vi "Exo5.vi"() -> ()   [LabVIEW 2018]
panel:
  in  "stop":bool
  in  "Débit":dbl
  out "Tank 2":dbl(slide) scale=0.0..3000.0
  in  "Consigne":dbl
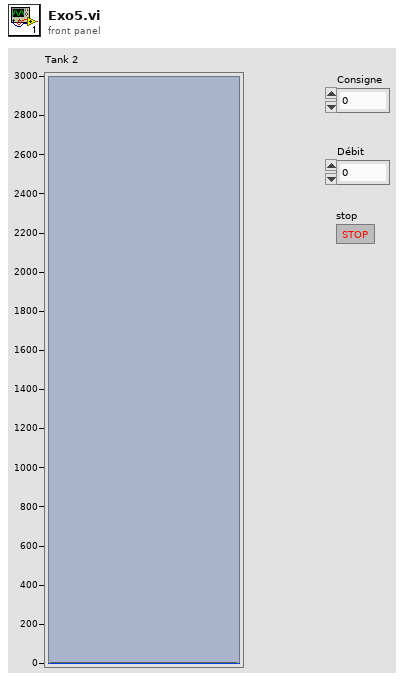
[diagram p1: front panel]
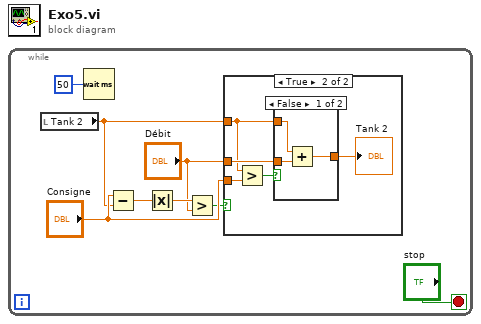
[diagram p0: block diagram]
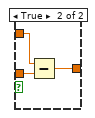
[diagram p3: hidden frame]
diagram:
  n1 = while {
    stop <- "stop" stop-if-true
    n2 = local read "Tank 2"() -> (w1:dbl)
    n3 = Wait (ms)(milliseconds to wait=u32 50) -> ()  [unwired: 1 out]
    n4 = Subtract(x="Consigne", y=w1) -> (x-y=w6:dbl)
    n5 = Absolute Value(x=w6) -> (abs(x)=w3:dbl)
    n6 = Greater?(x=w3, y="Débit") -> (0:w4:bool)
    n7 = case shown="True" w4 {
      tunnel: "Consigne" -> [_ w11]
      tunnel: "Débit" -> [_ w10]
      tunnel: w1 -> [_ w9]
      frame False {
      }
      frame True {
        n8 = Greater?(x=w9, y=w11) -> (0:w13:bool)
        n9 = case shown="False" w13 {
          tunnel: [w14 w19] -> w12
          tunnel: w9 -> [w16 w18]
          tunnel: w10 -> [w15 w17]
          frame False {
            n10 = Add(x=w16, y=w15) -> (x+y=w14:dbl)
          }
          frame True {
            n11 = Subtract(x=w18, y=w17) -> (x-y=w19:dbl)
          }
        }
        "Tank 2" <- w12
      }
    }
  }
